vi "Main.vi"() -> ()   [LabVIEW 2019]
doc: "The myRIO Project template acquires acceleration data from the onboard accelerometer and displays the changes of acceleration values in a waveform chart."
uses:
  <vilib>/Platform/TimedLoop/XDataNode/timing_clust.ctl
  <vilib>/Platform/TimedLoop/XDataNode/nitl_modes.ctl
  <vilib>/Platform/TimedLoop/XDataNode/wakeup.ctl
  <vilib>/myRIO/Instrument Drivers/Onboard IO/UART/typedef/VISA Configuration.ctl
  <vilib>/myRIO/Common/Instrument Driver Framework/myRIO v1.0/Encoder/typedefs/Encoder Signal Mode.ctl
  <vilib>/myRIO/Instrument Drivers/Onboard IO/Encoder/typedefs/Encoder Reference.ctl
  <vilib>/myRIO/Common/Instrument Driver Framework/Utilities/typedefs/myRIO Generic Hardware Reference.ctl
  <vilib>/myRIO/Common/Instrument Driver Framework/Utilities/typedefs/Hardware Version Enum.ctl
  <vilib>/myRIO/Common/Instrument Driver Framework/Utilities/typedefs/myRIO v1.0 Reference.ctl
  <vilib>/myRIO/Common/Instrument Driver Framework/Utilities/typedefs/Generic FPGA Reference.ctl
  <vilib>/myRIO/Common/Instrument Driver Framework/myRIO v1.0/Encoder/typedefs/Encoder Channels Enum.ctl
  <vilib>/myRIO/Common/Instrument Driver Framework/myRIO v1.0/Encoder/typedefs/Encoder Configuration v1.0.ctl
  <vilib>/userDefined/High Color/nirio_resource_hc.ctl
  <vilib>/myRIO/Instrument Drivers/Onboard IO/PWM/typedefs/PWM Reference.ctl
  <vilib>/myRIO/Common/Instrument Driver Framework/myRIO v1.0/PWM/typedefs/PWM Channels Enum.ctl
  <vilib>/myRIO/Instrument Drivers/Onboard IO/PWM/typedefs/PWM Configuration.ctl
  <vilib>/myRIO/Instrument Drivers/Onboard IO/DIO/typedefs/DIO Reference.ctl
  <vilib>/myRIO/Common/Instrument Driver Framework/myRIO v1.0/DIO/typedefs/DIO Channels List.ctl
  <vilib>/myRIO/Common/Instrument Driver Framework/myRIO v1.0/DIO/typedefs/DIO Channels Enum.ctl
  <vilib>/myRIO/Common/Instrument Driver Framework/Utilities/vis/Is FPGA Ref Available.vi
  <vilib>/myRIO/Common/Instrument Driver Framework/myRIO v1.0/Encoder/vis/myRIO v1.1 Open Encoder.vi
  <vilib>/myRIO/Instrument Drivers/Onboard IO/Encoder/vis/Read.vi
  <vilib>/myRIO/Common/Instrument Driver Framework/myRIO v1.0/PWM/vis/myRIO v1.1 Open PWM.vi
  <vilib>/myRIO/Common/Instrument Driver Framework/myRIO v1.0/DIO/vis/myRIO v1.1 Open DIO.vi
  <vilib>/myRIO/Instrument Drivers/Onboard IO/DIO/vis/Write.vi
  <vilib>/myRIO/Common/Instrument Driver Framework/myRIO v1.0/UART/vis/myRIO v1.0 Close UART.vi
  <vilib>/myRIO/Common/Instrument Driver Framework/Utilities/vis/Validate Channels.vi
  <vilib>/myRIO/Common/Instrument Driver Framework/myRIO v1.0/Encoder/vis/myRIO v1.0 Reserve Encoder.vi
  <vilib>/myRIO/Common/Instrument Driver Framework/myRIO v1.0/PWM/vis/myRIO v1.0 Reserve PWM.vi
  <vilib>/myRIO/Common/Instrument Driver Framework/myRIO v1.0/DIO/vis/myRIO v1.0 Reserve DIO.vi
  <vilib>/myRIO/Common/Instrument Driver Framework/myRIO v1.0/Encoder/vis/myRIO v1.0 Build MUX Configuration Encoder.vi
  <vilib>/myRIO/Common/Instrument Driver Framework/myRIO v1.0/Resource Manager/vis/myRIO v1.0 Reserve Channel List.vi
  <vilib>/myRIO/Common/Instrument Driver Framework/myRIO v1.0/PWM/vis/myRIO v1.0 Build MUX Configuration PWM.vi
  <vilib>/myRIO/Common/Instrument Driver Framework/myRIO v1.0/DIO/vis/myRIO v1.0 Build MUX Configuration DIO.vi
  <vilib>/myRIO/Common/Instrument Driver Framework/myRIO v1.0/Resource Manager/vis/myRIO v1.0 Create Configuration List.vi
  <vilib>/myRIO/Common/Instrument Driver Framework/myRIO v1.0/Resource Manager/vis/myRIO v1.0 Reserve Channel.vi
  <vilib>/myRIO/Common/Instrument Driver Framework/myRIO v1.0/Resource Manager/vis/myRIO v1.0 Unreserve Channel.vi
  <vilib>/myRIO/Common/Instrument Driver Framework/myRIO v1.0/Resource Manager/vis/myRIO v1.0 Build Mutex Name.vi
  <vilib>/Utility/VariantDataType/GetNumericInfo.vi
  <vilib>/Utility/error.llb/Error Cluster From Error Code.vi
  <vilib>/myRIO/Common/Instrument Driver Framework/myRIO v1.0/myRIO v1.1 Open.vi
  <vilib>/myRIO/Common/Instrument Driver Framework/Utilities/vis/IO Manager.vi
  <vilib>/myRIO/Common/Instrument Driver Framework/Utilities/vis/Configuration Manager.vi
  <vilib>/myRIO/Common/Instrument Driver Framework/myRIO v1.0/Resource Manager/vis/myRIO v1.0 Configure IO.vi
  <vilib>/myRIO/Common/Instrument Driver Framework/myRIO v1.0/myRIO v1.0 Close.vi
  <vilib>/myRIO/Common/Instrument Driver Framework/myRIO v1.0/Encoder/vis/myRIO v1.0 Configure Encoder.vi
  <vilib>/myRIO/Common/Instrument Driver Framework/myRIO v1.0/Encoder/vis/myRIO v1.0 Read Encoder.vi
  <vilib>/Utility/inputDevices.llb/joystickAcquire.vi
  <vilib>/myRIO/Common/Instrument Driver Framework/myRIO v1.0/PWM/vis/myRIO v1.0 Write PWM.vi
  <vilib>/myRIO/Common/Instrument Driver Framework/myRIO v1.0/DIO/vis/myRIO v1.0 Write DIO.vi
  <vilib>/Instr/_visa.llb/VISA Configure Serial Port (Instr).vi
  <vilib>/myRIO/Common/Instrument Driver Framework/Utilities/vis/FPGA Ref Manager.vi
  <vilib>/myRIO/Common/Instrument Driver Framework/myRIO v1.0/myRIO v1.0 Reset FPGA.vi
  <vilib>/myRIO/Common/Instrument Driver Framework/myRIO v1.0/IRQ/vis/myRIO v1.0 IRQ Info FGV.vi
  <vilib>/myRIO/Common/Instrument Driver Framework/myRIO v1.0/IRQ/vis/myRIO v1.0 Timer IRQ Info FGV.vi
  <vilib>/myRIO/Common/Instrument Driver Framework/myRIO v1.0/IRQ/vis/myRIO v1.0 ISR Agent.vi
  <vilib>/myRIO/Instrument Drivers/Utilities/vis/Reset Index.vi
  <vilib>/myRIO/Common/Instrument Driver Framework/myRIO v1.0/Resource Manager/vis/myRIO v1.0 Block Write Resource Manager.vi
  <vilib>/platform/TimedLoop/XDataNode/XDataNode.xnode
  <vilib>/myRIO/Express VI/Onboard IO/Encoder/Encoder Express VI.xnode
  <vilib>/myRIO/Instrument Drivers/Onboard IO/Encoder/vis/myRIO Encoder Open.xnode
  <vilib>/myRIO/Common/Instrument Driver Framework/myRIO v1.0/Encoder/typedefs/Encoder Count Direction Enum.ctl
  <vilib>/myRIO/Express VI/Onboard IO/PWM/PWM Express VI.xnode
  <vilib>/myRIO/Instrument Drivers/Onboard IO/PWM/vis/myRIO PWM Open.xnode
  <vilib>/myRIO/Express VI/Onboard IO/DO/DO Express VI.xnode
  <vilib>/myRIO/Instrument Drivers/Onboard IO/DIO/vis/myRIO DIO Open.xnode
  <vilib>/myRIO/Express VI/Onboard IO/UART/UART Express VI.xnode
  <vilib>/Platform/TimedLoop/XDataNode/XDNodeRunTimeDep.lvlib
  <vilib>/myRIO/Instrument Drivers/Onboard IO/Encoder/Encoder.lvlib
  <vilib>/myRIO/Instrument Drivers/Onboard IO/PWM/PWM.lvlib
  <vilib>/myRIO/Instrument Drivers/Onboard IO/DIO/DIO.lvlib
  <vilib>/myRIO/Instrument Drivers/Utilities/Utilities.lvlib
  <vilib>/myRIO/Instrument Drivers/Onboard IO/UART/UART.lvlib
panel:
  in  "kill switch":bool
  out "reverse":bool
  out "button 2":bool
  out "button 3":bool
  out "stop":bool
  out "pov 1":i32
  out "X axis":i32
  out "Gauge":dbl(knob) scale=0.0..2500.0
  out "Counter Value":i32
  out "x*y":dbl
  out "Y axis":i32
  out "Z axis rotation":i32
  out "x >= 0?":bool
  out "x/y 2":dbl
  out "x*y 2":dbl
  out "x >= y?":bool
  out "abs(x)":dbl
  out "Numeric Control":dbl
  out "x-y":dbl
  out "button 1":bool
  out "x/y 3":dbl
  out "x <= 0?":bool
  out "Numeric Control 4":dbl
  out "Numeric Control 3":dbl
  out "Character Count":u32
  out "x/y 4":dbl
  out "resulting string":string
  in  "device index":i32
  in  "[ESC]":bool
  out "pulse width [ms]":dbl=1.5
  out "duty cycle [%]":dbl
  in  "null offset":bool
  out "offset [%FS]":dbl
  out "x/y":dbl
  in  "PWM channel":tag="B/PWM0"
  in  "device index 2":i32
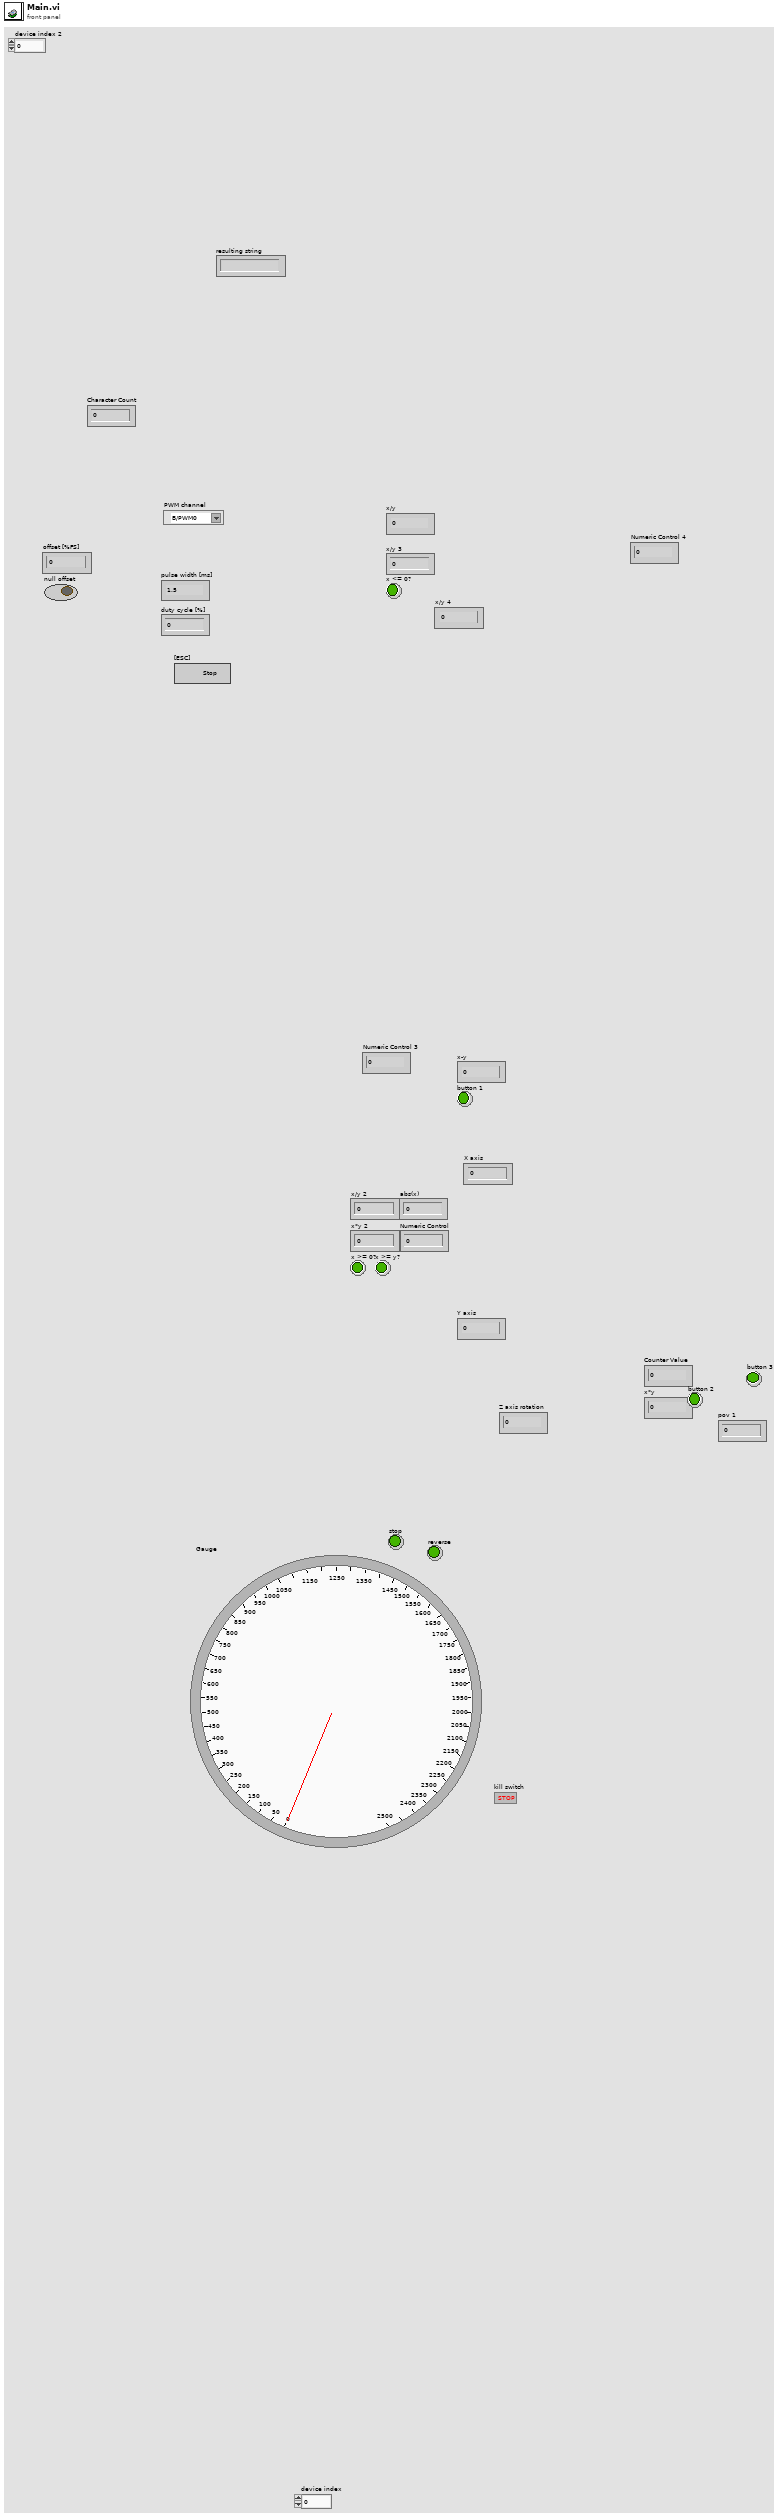
[diagram p1: front panel]
types:
  T1 = typedef "XDNodeRunTimeDep.lvlib/timing_clust.ctl" = cluster{"Expected End [f-1]":u64, "Actual End [f-1]":u64, "Finished Late? [f-1]":bool, "Expected End [i-1]":u64, "Actual End [i-1]":u64, "Finished Late? [i-1]":bool, "Expected Start [i]":u64, "Actual Start [i]":u64, "Expected Start [f]":u64, "Actual Start [f]":u64, "Source Name":string, "Structure Name":string, "Period":i64, "Deadline":i64, "Offset":i64, "Start":i64, "Priority":i32, "Timeout":i32, "Mode":T2, "Wakeup Reason":T3, "Error":errorcluster, "Source Type":string, "Secondary Source Type":string, "Global End Time":u64, "Global Start Time":u64, "Frame Duration":u64, "Iteration Duration":u64, "Assigned CPU":i32, "I/O Scan Engine Mode":u32}
  T2 = typedef "XDNodeRunTimeDep.lvlib/nitl_modes.ctl" = enum32{"No Change", "Process missed periods, maintain original phase", "Discard missed periods, maintain original phase", "Process missed periods, ignore original phase", "Discard missed periods, ignore original phase"}
  T3 = typedef "XDNodeRunTimeDep.lvlib/wakeup.ctl" = enum32{"Normal", "Aborted", "Asynchronous wakeup", "Timing source error", "Timed loop error", "Timeout"}
  T4 = typedef "UART.lvlib/VISA Configuration.ctl" = cluster{"baud rate (9600)":u32, "data bits (8)":u16, "parity (0:none)":enum16{"None", "Odd", "Even", "Mark", "Space"}, "stop bits (10: 1 bit)":u16, "flow control (0:none)":u16, "termination char\n(0xA = '\\n' = LF) ":u8, "Enable Termination\nChar (T)":bool, "timeout (10sec)":u32}
  T5 = typedef "DIO.lvlib/DIO Reference.ctl" = cluster{"myRIO Reference":T6, "DIO Channels List":T10}
  T6 = typedef "myRIO Generic Hardware Reference.ctl" = cluster{"myRIO Model":T7, "myRIO Hardware Reference":T8}
  T7 = typedef "Hardware Version Enum.ctl" = enum16{"Unknown", "myRIO-1900", "myRIO-1950", "roboRIO", "NI ELVIS RIO CM", "ELVIS III"}
  T8 = typedef "myRIO v1.0 Reference.ctl" = cluster{"Generic FPGA Reference":T9, "Allow multiple opens":bool}
  T9 = typedef "Generic FPGA Reference.ctl" = refnum<k20>
  T10 = typedef "DIO Channels List.ctl" = T11[]
  T11 = typedef "DIO Channels Enum.ctl" = enum16{"Not Connected", "C/DIO0", "C/DIO1", "C/DIO2", "C/DIO3", "C/DIO4", "C/DIO5", "C/DIO6", "C/DIO7", "A/DIO0", "A/DIO1", "A/DIO2", "A/DIO3", "A/DIO4", "A/DIO5", "A/DIO6", "A/DIO7", "A/DIO8", "A/DIO9", "A/DIO10", "A/DIO11", "A/DIO12", "A/DIO13", "A/DIO14", "A/DIO15", "A/DIO16", "A/DIO17", "A/DIO18", "A/DIO19", "B/DIO0", "B/DIO1", "B/DIO2", "B/DIO3", "B/DIO4", "B/DIO5", "B/DIO6", "B/DIO7", "B/DIO8", "B/DIO9", "B/DIO10", "B/DIO11", "B/DIO12", "B/DIO13", "B/DIO14", "B/DIO15", "B/DIO16", "B/DIO17", "B/DIO18", "B/DIO19", "LED0", "LED1", "LED2", "LED3", "Button0", "DIO/DIO0", "DIO/DIO1", "DIO/DIO2", "DIO/DIO3", "DIO/DIO4", "DIO/DIO5", "DIO/DIO6", "DIO/DIO7", "DIO/DIO8", "DIO/DIO9", "SPI/CS0", "SPI/CS1", "SPI/CS2", "SPI/CS3", "LED RADIO (Green)", "LED RADIO (Red)", "LED COMM (Green)", "LED COMM (Red)", "LED MODE (Green)", "LED MODE (Red)"}
  T12 = typedef "nirio_resource_hc.ctl" = tag
  T13 = typedef "PWM.lvlib/PWM Reference.ctl" = cluster{"myRIO Reference":T6, "PWM Channels Enum":T14, "PWM Configuration":T15}
  T14 = typedef "PWM Channels Enum.ctl" = enum16{"Not Connected", "C/PWM0", "C/PWM1", "A/PWM0", "A/PWM1", "A/PWM2", "A/PWM3", "A/PWM4", "A/PWM5", "A/PWM6", "A/PWM7", "A/PWM8", "A/PWM9", "A/PWM10", "A/PWM11", "A/PWM12", "A/PWM13", "A/PWM14", "A/PWM15", "A/PWM16", "A/PWM17", "A/PWM18", "A/PWM19", "B/PWM0", "B/PWM1", "B/PWM2", "B/PWM3", "B/PWM4", "B/PWM5", "B/PWM6", "B/PWM7", "B/PWM8", "B/PWM9", "B/PWM10", "B/PWM11", "B/PWM12", "B/PWM13", "B/PWM14", "B/PWM15", "B/PWM16", "B/PWM17", "B/PWM18", "B/PWM19", "PWM/PWM0", "PWM/PWM1", "PWM/PWM2", "PWM/PWM3", "PWM/PWM4", "PWM/PWM5", "PWM/PWM6", "PWM/PWM7", "PWM/PWM8", "PWM/PWM9"}
  T15 = typedef "PWM.lvlib/PWM Configuration.ctl" = cluster{"Frequency":dbl, "Duty Cycle":dbl}
  T16 = typedef "Encoder.lvlib/Encoder Reference.ctl" = cluster{"myRIO Reference":T6, "Encoder Channels Enum":T17}
  T17 = typedef "Encoder Channels Enum.ctl" = enum16{"Not Connected", "C/ENC0", "C/ENC1", "A/ENC", "A/ENC0", "A/ENC1", "A/ENC2", "A/ENC3", "A/ENC4", "A/ENC5", "A/ENC6", "A/ENC7", "A/ENC8", "A/ENC9", "B/ENC", "B/ENC0", "B/ENC1", "B/ENC2", "B/ENC3", "B/ENC4", "B/ENC5", "B/ENC6", "B/ENC7", "B/ENC8", "B/ENC9", "DIO/ENC0", "DIO/ENC1", "DIO/ENC2", "DIO/ENC3", "DIO/ENC4"}
  T18 = typedef "Encoder Signal Mode.ctl" = enum16{"Quadrature phase signal", "Step and direction signal"}
  T19 = cluster{"X axis":i32, "Y axis":i32, "Z axis":i32, "X axis rotation":i32, "Y axis rotation":i32, "Z axis rotation":i32, "U axis":i32, "V axis":i32}
  T20 = cluster{"button 1":bool, "button 2":bool, "button 3":bool, "button 4":bool, "button 5":bool, "button 6":bool, "button 7":bool, "button 8":bool, "button 9":bool, "button 10":bool, "button 11":bool, "button 12":bool, "button 13":bool, "button 14":bool, "button 15":bool, "button 16":bool, "button 17":bool, "button 18":bool, "button 19":bool, "button 20":bool, "button 21":bool, "button 22":bool, "button 23":bool, "button 24":bool, "button 25":bool, "button 26":bool, "button 27":bool, "button 28":bool, "button 29":bool, "button 30":bool, "button 31":bool, "button 32":bool}
  T21 = cluster{"pov 1":i32, "pov 2":i32, "pov 3":i32, "pov 4":i32}
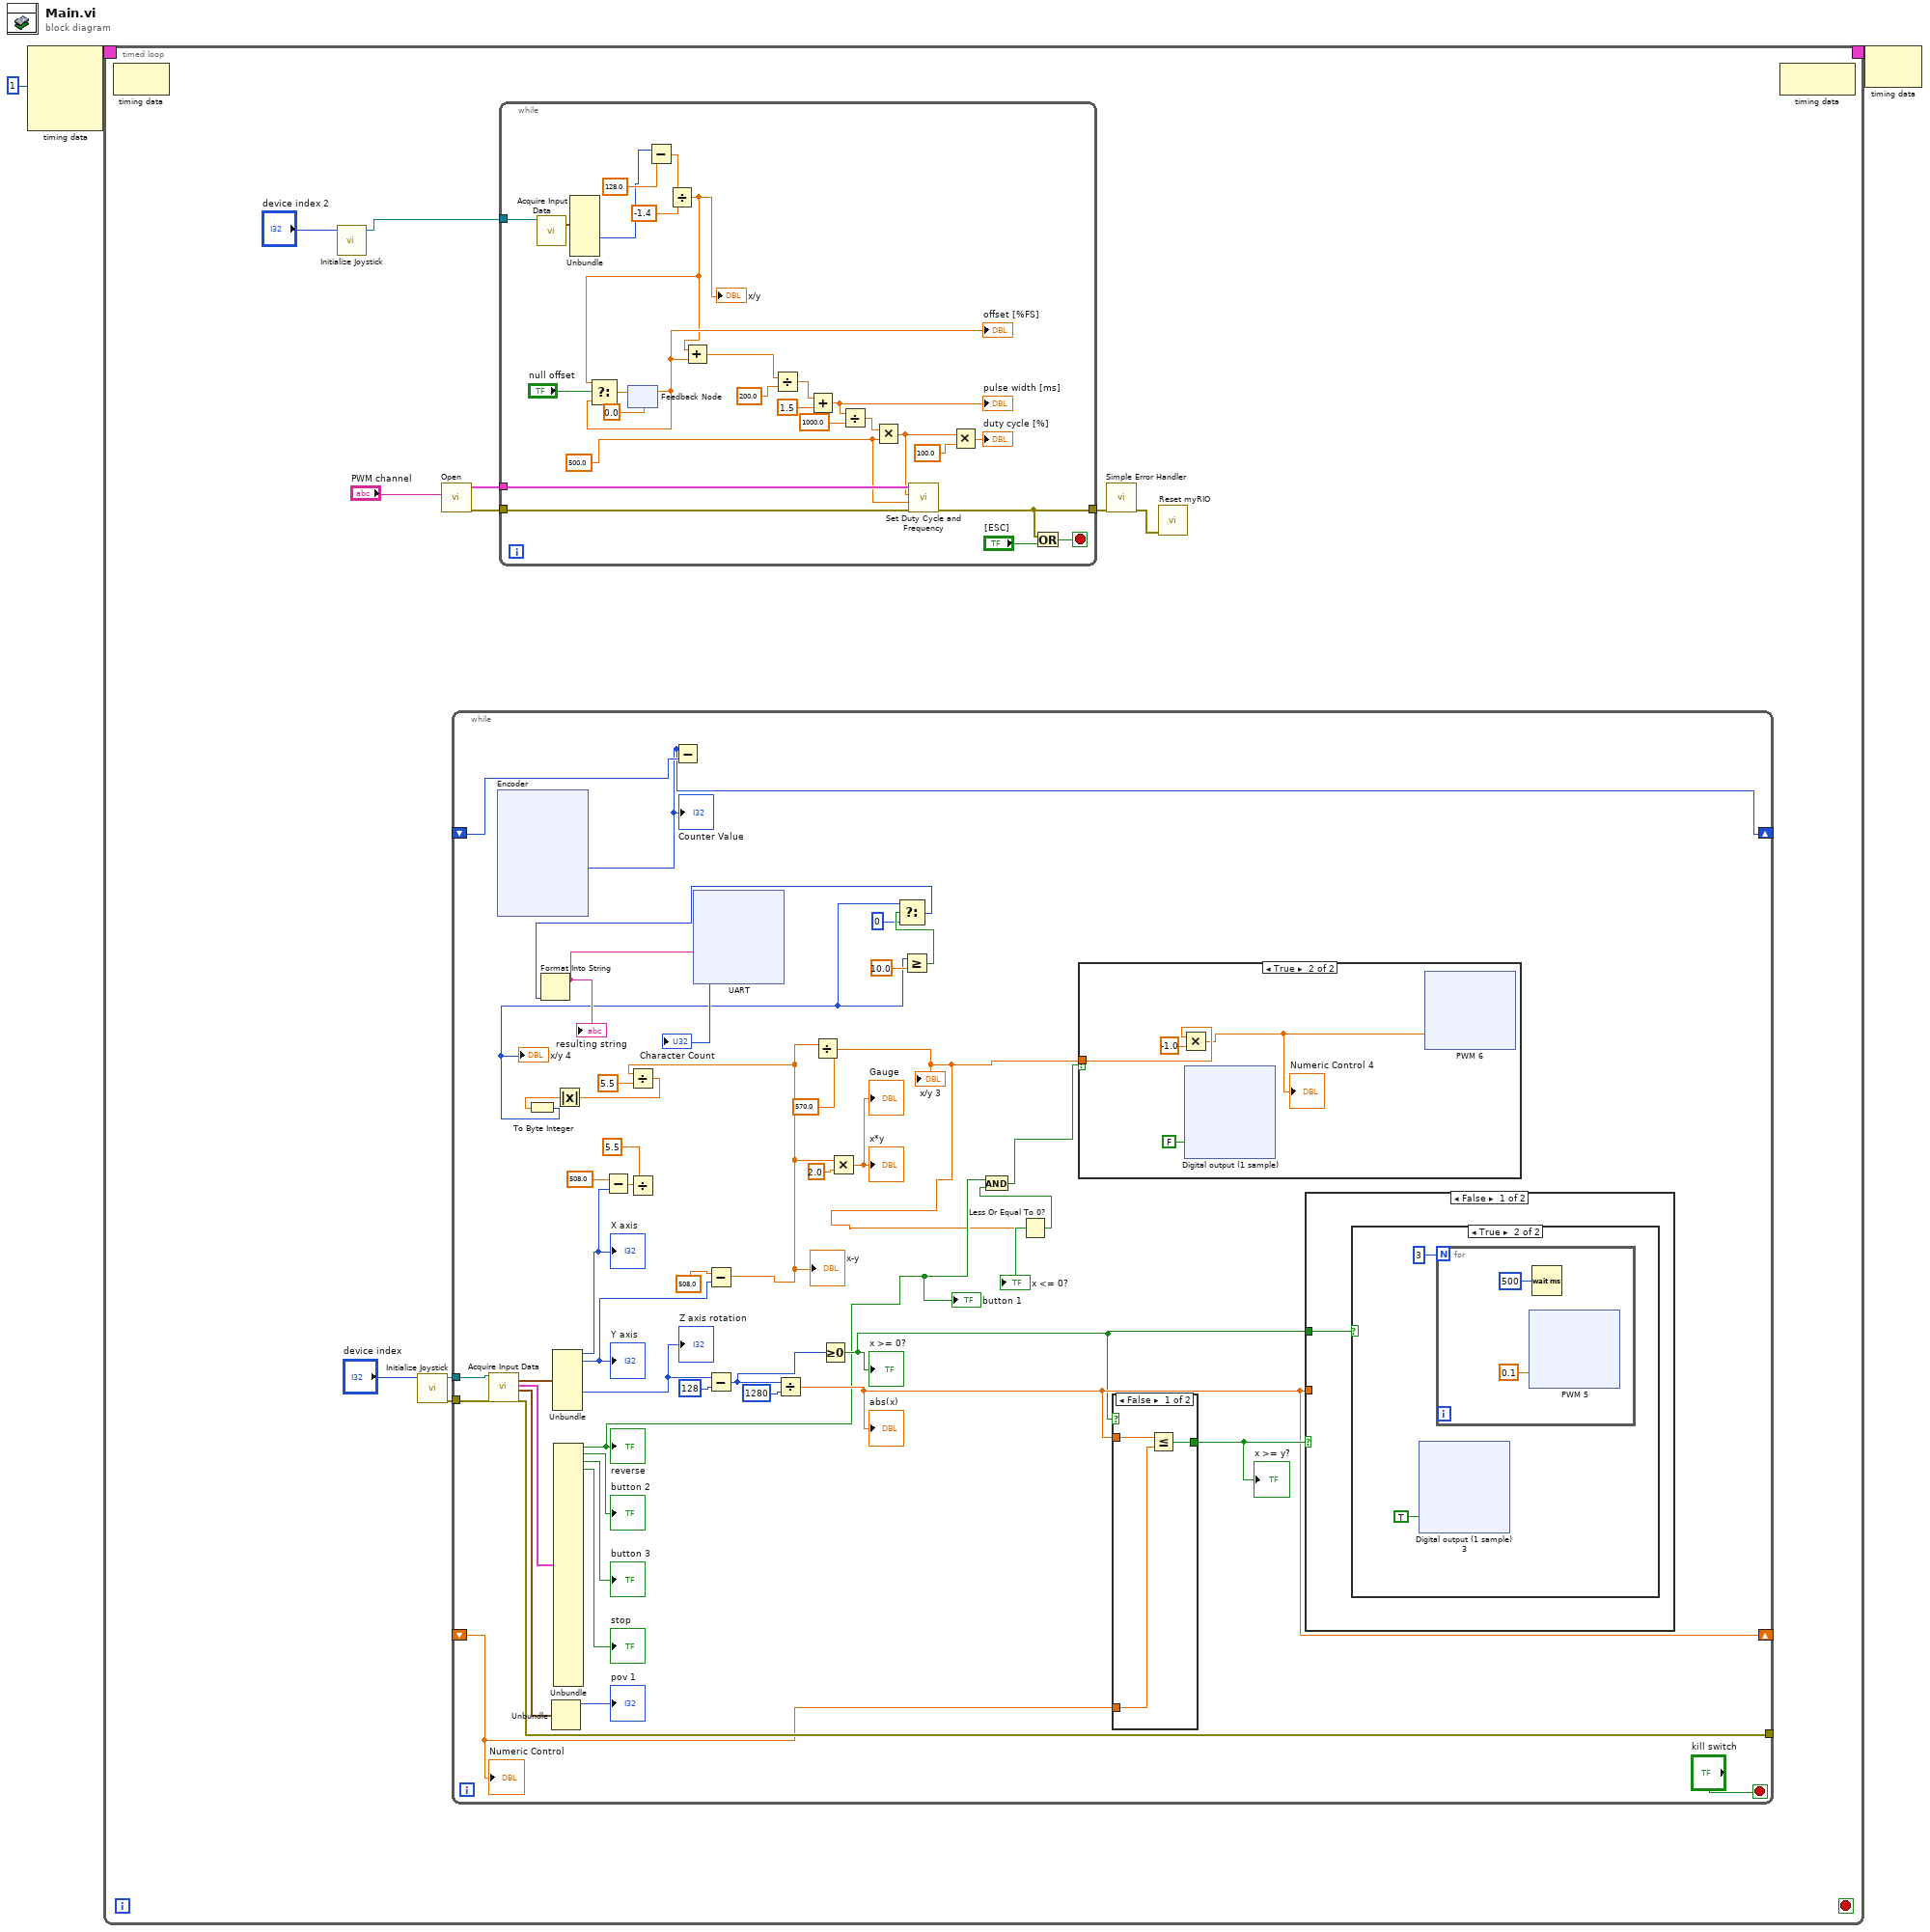
[diagram p0: block diagram]
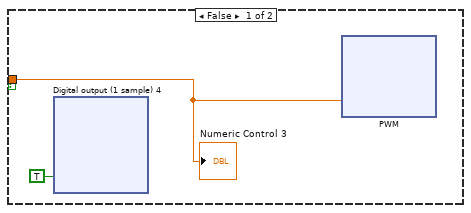
[diagram p2: hidden frame]
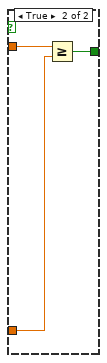
[diagram p3: hidden frame]
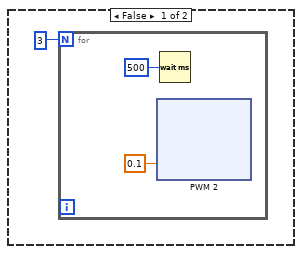
[diagram p4: hidden frame]
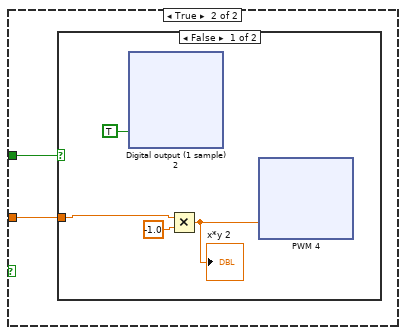
[diagram p5: hidden frame]
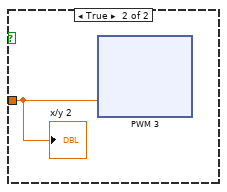
[diagram p6: hidden frame]
diagram:
  n1 = node-c288(i64 1 ("Period")) -> (w3:T1)  [unwired: 3 in]
  n2 = timed-loop {
    timing: w3 -> [_]
    timing-out: [_] -> w2
    stop <- _ stop-if-true
    n3 = node-c288() -> ()  [unwired: 1 in, 1 out]
    n4 = call <vilib>:"Initialize Joystick.vi"("device index"="device index 2") -> ("device ID"=w4:refnum<k1>)  [unwired: 9 in, 1 out]
    n5 = call <vilib>:"Initialize Joystick.vi"("device index"="device index") -> ("error out"=w11:errorcluster, "device ID"=w12:refnum<k1>)  [unwired: 9 in]
    n6 = call <vilib>:"Open.vi"("Channel Name"="PWM channel") -> ("error out"=w7:errorcluster, "PWM Ref Out"=w8:T13)  [unwired: 9 in]
    n7 = while {
      tunnel: w12 -> [w85]
      tunnel: w11 -> [w84]
      tunnel: [w83] -> _
      shift-right: [w56] -> _
      shift-left: _ -> [w78]
      shift-right: [w64] -> _
      shift-left: _ -> [w66]
      stop <- "kill switch" stop-if-true
      n8 = call-poly <vilib>:"Acquire Input Data.vi"("device ID"=w85, "error in (no error)"=w84) -> ("axis info"=w73:T19, "button info"=w82:T20, "direction info"=w80:T21, "error out"=w83:errorcluster)  [unwired: 13 in, 1 out]
      n9 = xnode "Encoder"() -> ("Counter Value"=w56:i32)  [unwired: 2 in, 3 out]
      "Counter Value" <- w56
      n10 = Unbundle(w80) -> ("pov 1"=→"pov 1":i32)  [unwired: 3 out]
      n11 = Unbundle(w73) -> ("X axis"=w59:i32, "Y axis"=w62:i32, "Z axis rotation"=w68:i32)  [unwired: 5 out]
      "X axis" <- w59
      "Y axis" <- w62
      "Z axis rotation" <- w68
      n12 = Unbundle(w82) -> ("button 1"=w54:bool, "button 2"=→"button 2":bool, "button 3"=→"button 3":bool, "button 4"=→"stop":bool)  [unwired: 28 out]
      "reverse" <- w54
      "button 1" <- w54
      n13 = Subtract(x=508.0, y=w59) -> (x-y=w58:dbl)
      n14 = Divide(x=w58, y=5.5) -> ()  [unwired: 1 out]
      n15 = Subtract(x=w56, y=w78) -> ()  [unwired: 1 out]
      n16 = Subtract(x=508.0 ("y"), y=w62) -> (x-y=w48:dbl)
      "x-y" <- w48
      n17 = Divide(x=w48, y=5.5) -> (x/y=w47:dbl)
      n18 = Absolute Value(x=w47) -> (abs(x)=w46:dbl)
      n19 = To Byte Integer(number=w46) -> (8bit integer=w43:i8)
      "x/y 4" <- w43
      n20 = Subtract(x=w68, y=128) -> (x-y=w67:i32)
      n21 = Divide(x=w67, y=1280) -> (x/y=w64:dbl)
      "abs(x)" <- w64
      n22 = Divide(x=w48, y=570.0) -> (x/y=w50:dbl)
      "x/y 3" <- w50
      n23 = Greater Or Equal To 0?(x=w67) -> (x >= 0?=w63:bool)
      "x >= 0?" <- w63
      n24 = Multiply(x=w48, y=2.0) -> (x*y=→"Gauge" →"x*y":dbl)
      n25 = Greater Or Equal?(x=w43, y=10.0) -> (x >= y?=w44:bool)
      n26 = Select(t=w43, s=w44, f=i8 0) -> (s? t:f=w41:i8)
      n27 = Format Into String "Format Into String"(w41) -> (resulting string=w51:string)  [unwired: 3 in, 1 out]
      "resulting string" <- w51
      n28 = xnode "UART"("Characters to Write"=w51) -> ("Character Count"=→"Character Count":u32)  [unwired: 1 in, 1 out]
      n29 = Less Or Equal To 0?(x=w50) -> (x <= 0?=w55:bool)
      "x <= 0?" <- w55
      n30 = And(x=w54, y=w55) -> (x .and. y?=w53:bool)
      n31 = case shown="True" w53 {
        tunnel: w50 -> [w103 w176]
        frame False {
          n32 = xnode "Digital output (1 sample) 4"("A/DIO0 (Pin 11)"=TRUE) -> ()  [unwired: 1 in, 1 out]
          n33 = xnode "PWM"("Duty Cycle"=w103) -> ()  [unwired: 1 in, 1 out]
          "Numeric Control 3" <- w103
        }
        frame True {
          n34 = Multiply(x=w176, y=-1.0) -> (x*y=w175:dbl)
          "Numeric Control 4" <- w175
          n35 = xnode "Digital output (1 sample)"("A/DIO0 (Pin 11)"=FALSE) -> ()  [unwired: 1 in, 1 out]
          n36 = xnode "PWM 6"("Duty Cycle"=w175) -> ()  [unwired: 1 in, 1 out]
        }
      }
      n37 = case shown="False" w63 {
        tunnel: w66 -> [w250 w253]
        tunnel: [w248 w252] -> w65
        tunnel: w64 -> [w249 w251]
        frame False {
          n38 = Less Or Equal?(x=w249, y=w250) -> (x <= y?=w248:bool)
        }
        frame True {
          n39 = Greater Or Equal?(x=w251, y=w253) -> (x >= y?=w252:bool)
        }
      }
      "x >= y?" <- w65
      n40 = case shown="False" w65 {
        tunnel: w63 -> [w254 w368]
        tunnel: w64 -> [_ w367]
        frame False {
          n41 = case shown="True" w254 {
            frame False {
              n42 = for {
                N: 3 -> [_]
                n43 = xnode "PWM 2"("Duty Cycle"=0.1) -> ()  [unwired: 1 in, 1 out]
                n44 = Wait (ms)(milliseconds to wait=u32 500) -> ()  [unwired: 1 out]
              }
            }
            frame True {
              n45 = xnode "Digital output (1 sample) 3"("A/DIO0 (Pin 11)"=TRUE) -> ()  [unwired: 1 in, 1 out]
              n46 = for {
                N: 3 -> [_]
                n47 = xnode "PWM 5"("Duty Cycle"=0.1) -> ()  [unwired: 1 in, 1 out]
                n48 = Wait (ms)(milliseconds to wait=u32 500) -> ()  [unwired: 1 out]
              }
            }
          }
        }
        frame True {
          n49 = case shown="False" w368 {
            tunnel: w367 -> [w371 w443]
            frame False {
              n50 = xnode "Digital output (1 sample) 2"("A/DIO0 (Pin 11)"=TRUE) -> ()  [unwired: 1 in, 1 out]
              n51 = Multiply(x=w371, y=-1.0) -> (x*y=w369:dbl)
              "x*y 2" <- w369
              n52 = xnode "PWM 4"("Duty Cycle"=w369) -> ()  [unwired: 1 in, 1 out]
            }
            frame True {
              n53 = xnode "PWM 3"("Duty Cycle"=w443) -> ()  [unwired: 1 in, 1 out]
              "x/y 2" <- w443
            }
          }
        }
      }
      "Numeric Control" <- w66
    }
    n54 = while {
      tunnel: w8 -> [w33]
      tunnel: w7 -> [w32]
      tunnel: [w31] -> w6
      tunnel: w4 -> [w20]
      stop <- w40 stop-if-true
      w14 = 500.0 ("y")
      n55 = call-poly <vilib>:"Acquire Input Data.vi"("device ID"=w20) -> ("axis info"=w21:T19)  [unwired: 14 in, 4 out]
      n56 = Unbundle(w21) -> ("Z axis rotation"=w15:i32)  [unwired: 7 out]
      n57 = feedback #1(0.0 ("position [%FS]")) -> (w27:dbl)
      "offset [%FS]" <- w27
      n58 = Subtract(x=w15, y=128.0) -> (x-y=w19:dbl)
      n59 = Divide(x=w19, y=-1.4) -> (x/y=w17:dbl)
      "x/y" <- w17
      n60 = Select(t=w17, s="null offset", f=w27) -> (s? t:f=w29:dbl)
      n61 = feedback-in #1(w29) -> ()
      n62 = Add(x=w17, y=w27) -> (x+y=w28:dbl)
      n63 = Divide(x=w28, y=200.0) -> (x/y=w37:dbl)
      n64 = Add(x=w37, y=1.5) -> (x+y=w35:dbl)
      "pulse width [ms]" <- w35
      n65 = Divide(x=w35, y=1000.0) -> (x/y=w26:dbl)
      n66 = Multiply(x=w26, y=w14) -> (x*y=w23:dbl)
      n67 = call <vilib>:"Set Duty Cycle and Frequency.vi"("error in (no error)"=w32, "Frequency [Hz]"=w14, "Duty Cycle"=w23, "PWM Ref In"=w33) -> ("error out"=w31:errorcluster)  [unwired: 5 in, 1 out]
      n68 = Multiply(x=w23, y=100.0) -> (x*y=→"duty cycle [%]":dbl)
      n69 = Or(x=w31, y="[ESC]") -> (x .or. y?=w40:bool)
    }
    n70 = call <vilib>:"Simple Error Handler.vi"("error in (no error)"=w6) -> ("error out"=w10:errorcluster)  [unwired: 4 in, 4 out]
    n71 = call <vilib>:"Reset myRIO.vi"("error in (no error)"=w10) -> ()  [unwired: 10 in, 1 out]
    n72 = node-c288() -> ()  [unwired: 1 in, 1 out]
  }
  n73 = node-c288(w2) -> ()  [unwired: 1 out]
